vi "FPGAvi.vi"() -> ()   [LabVIEW 2009]
uses:
  Signal Options.ctl
  Sequence.ctl
  <vilib>/Platform/TimedLoop/XDataNode/XDataNode.xnode
  <vilib>/Platform/TimedLoop/XDataNode/loadlvalarms.vi
  <vilib>/Platform/TimedLoop/XDataNode/timing_clust.ctl
  <vilib>/Platform/TimedLoop/XDataNode/nitl_modes.ctl
  <vilib>/Platform/TimedLoop/XDataNode/wakeup.ctl
  <vilib>/eio/EIONode/EIONode.xnode
  <vilib>/rvi/eio/nirviEIOImplementation/nirviEIOImplementation.xnode
  <vilib>/rvi/eio/common/nirviEmuTemplateMethod_noerrors.vi
  <vilib>/rvi/eio/common/nirviEmuClasses.ctl
  <vilib>/Platform/TimedLoop/XDataNode/XDNodeRunTimeDep.lvlib
panel:
  out "t_last_chop+t_dark-t_off":u64
  out "T_last-chop + t_dark":u64
  out "T_last-chop":u64
  out "t_chop":u64
  out "Current State":T1
  in  "Memory Sequence Duration":u64=240000
  out "t_mem":u64
  in  "Repump Duration":u64
  in  "Pump Duration":u64
  in  "Trapping Duration":u64
  in  "Chopper Dark Time":u64=15200
  out "Output Trigger":bool
  out "Global Time":u64
  out "Memory Timer":u64
  in  "Time to Activate B":u64=120000
  in  "Memory Mode":T2=enum."Coherent Memory Sequence"
  in  "Optical Density Sign":bool
  in  "Optical Density - stop":u64
  in  "Optical Density - start":u64
  in  "DLCZ Sign":bool
  in  "DLCZ start":u64
  in  "DLCZ stop":u64
  in  "Generate DLCZ Pulses":bool
  in  "DLCZ Period":u32
  in  "Time to Cut B":u64=120000
  in  "Minimum Period Between Memory Sequences":u64=800000
  in  "Trigger on Slope":enum8{"either", "false-true", "true-false"}(ring)=enum."true-false"
  in  "Stop":bool
  out "Active":bool
  in  "Output Trigger Sign":bool
  in  "Signal Sign":bool
  in  "Control Sign":bool
  in  "Repetition Period":u32
  in  "Switch Trigger (Shift Decimation)":bool
  in  "Trigger Source":bool
  in  "Pulse Selection":bool=TRUE
  in  "Signal stop":u64
  in  "Control - stop":u64
  in  "Signal start":u64
  in  "Control - start":u64
  # "External"
  # "Internal"
  # "All Pulses"
  # "1 out of 2 Pulses"
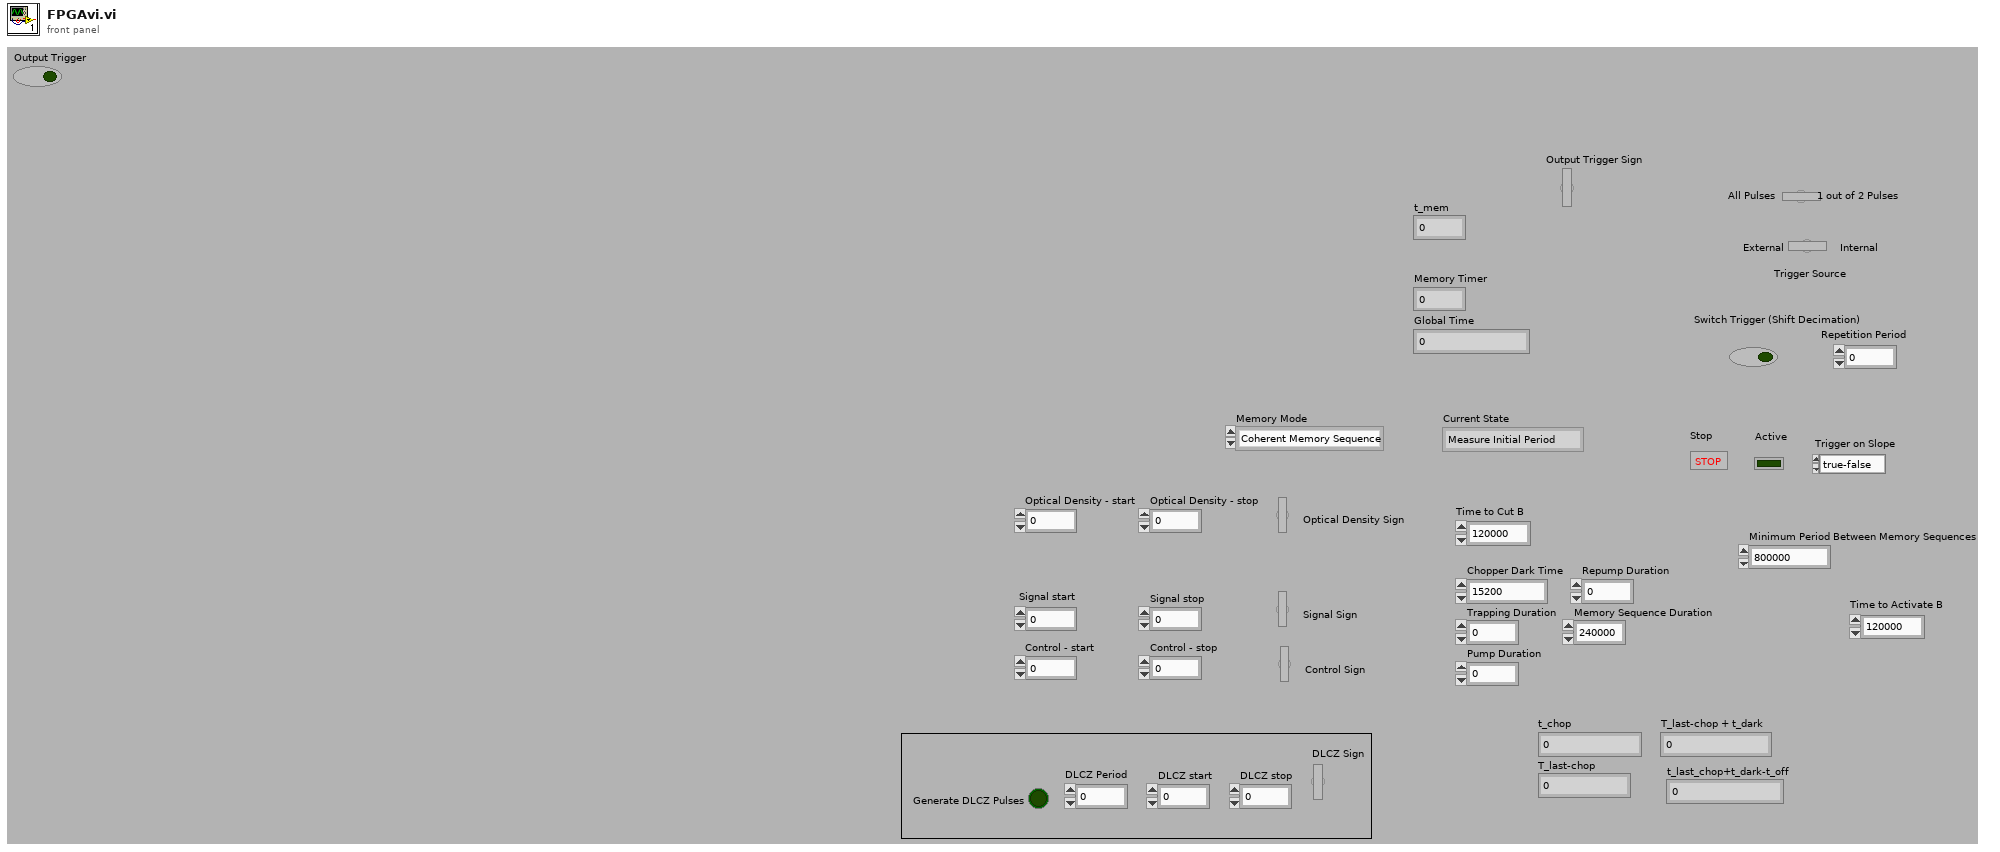
[diagram p1: front panel]
types:
  T1 = typedef "Sequence.ctl" = enum16{"Measure Initial Period", "Build MOT", "Wait for Deactivate Signal", "Deactivate B field", "Memory Sequence"}
  T2 = typedef "Signal Options.ctl" = enum16{"Generate DLCZ Pulses", "Measure Optical Density", "Coherent Memory Sequence", "Squeezed Memory Sequence"}
  T3 = typedef "XDNodeRunTimeDep.lvlib/timing_clust.ctl" = cluster{"Expected End [f-1]":u64, "Actual End [f-1]":u64, "Finished Late? [f-1]":bool, "Expected End [i-1]":u64, "Actual End [i-1]":u64, "Finished Late? [i-1]":bool, "Expected Start [i]":u64, "Actual Start [i]":u64, "Expected Start [f]":u64, "Actual Start [f]":u64, "Source Name":string, "Structure Name":string, "Period":i64, "Deadline":i64, "Offset":i64, "Start":i64, "Priority":i32, "Timeout":i32, "Mode":T4, "Wakeup Reason":T5, "Error":errorcluster, "Source Type":string, "Secondary Source Type":string, "Global End Time":u64, "Global Start Time":u64, "Frame Duration":u64, "Iteration Duration":u64, "Assigned CPU":i32, "I/O Scan Engine Mode":u32}
  T4 = typedef "XDNodeRunTimeDep.lvlib/nitl_modes.ctl" = enum32{"No Change", "Process missed periods, maintain original phase", "Discard missed periods, maintain original phase", "Process missed periods, ignore original phase", "Discard missed periods, ignore original phase"}
  T5 = typedef "XDNodeRunTimeDep.lvlib/wakeup.ctl" = enum32{"Normal", "Aborted", "Asynchronous wakeup", "Timing source error", "Timed loop error", "Timeout"}
  T6 = typedef "nirviEmuClasses.ctl" = enum16{"IO Read", "IO Write", "Method", "Property Read", "Property Write"}
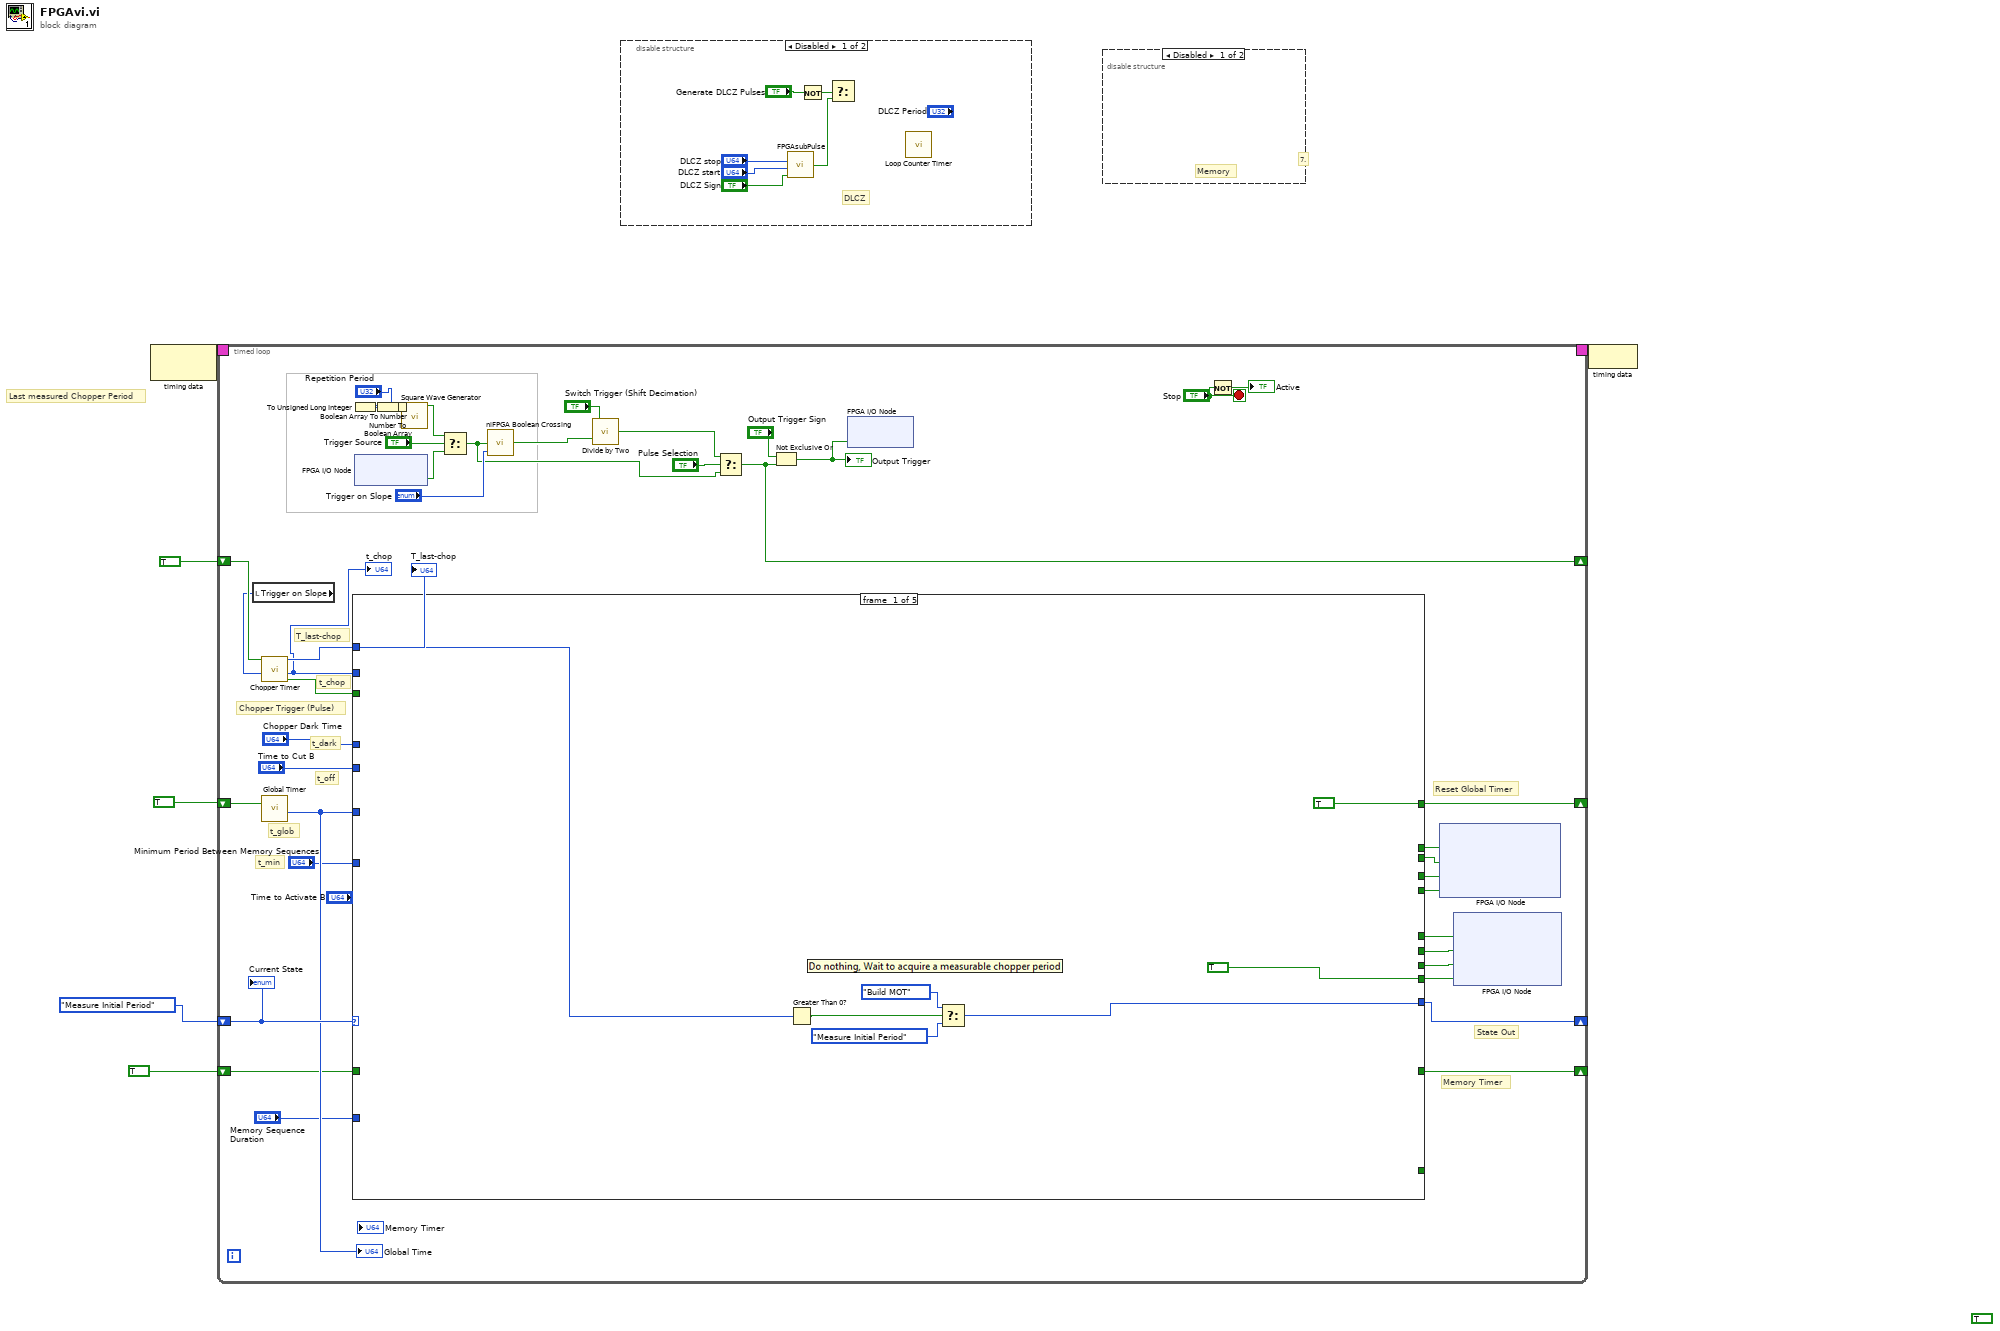
[diagram p0: block diagram]
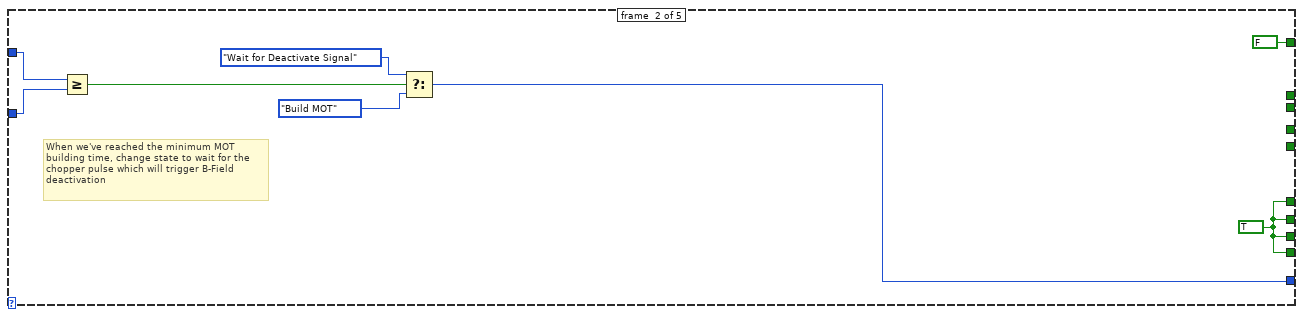
[diagram p4: hidden frame]
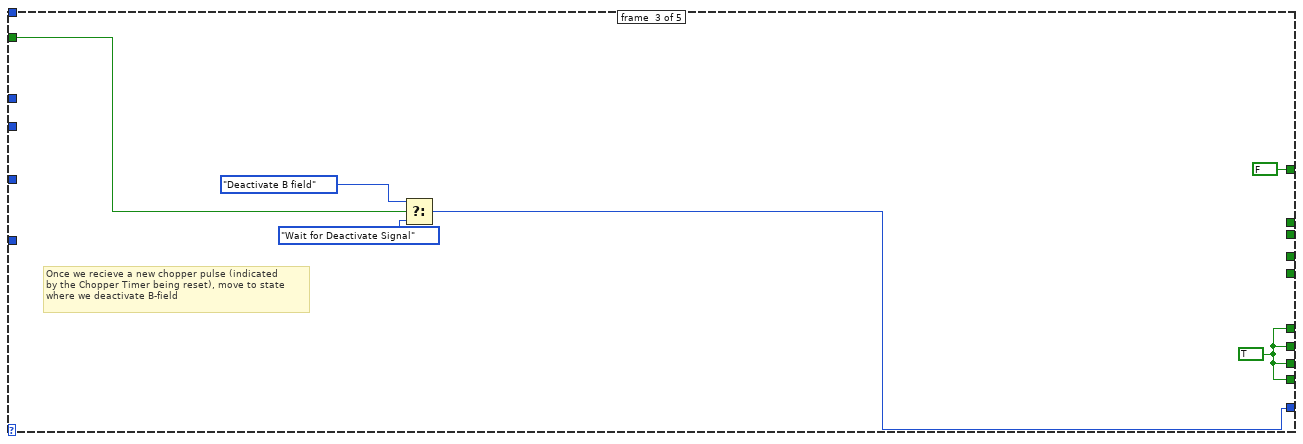
[diagram p5: hidden frame]
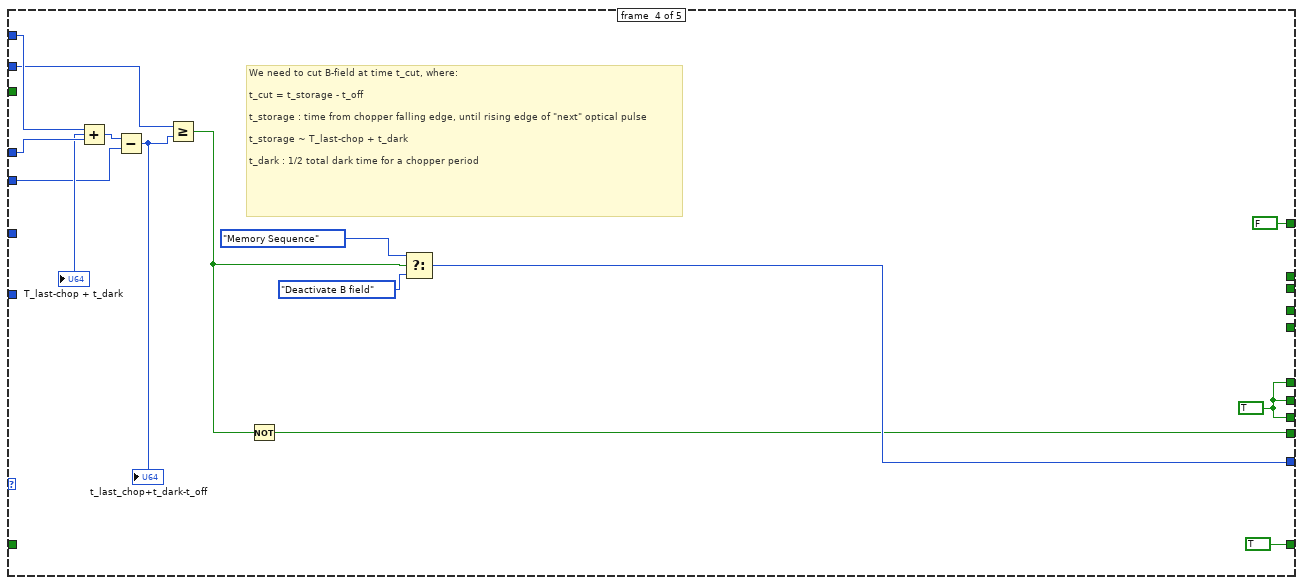
[diagram p6: hidden frame]
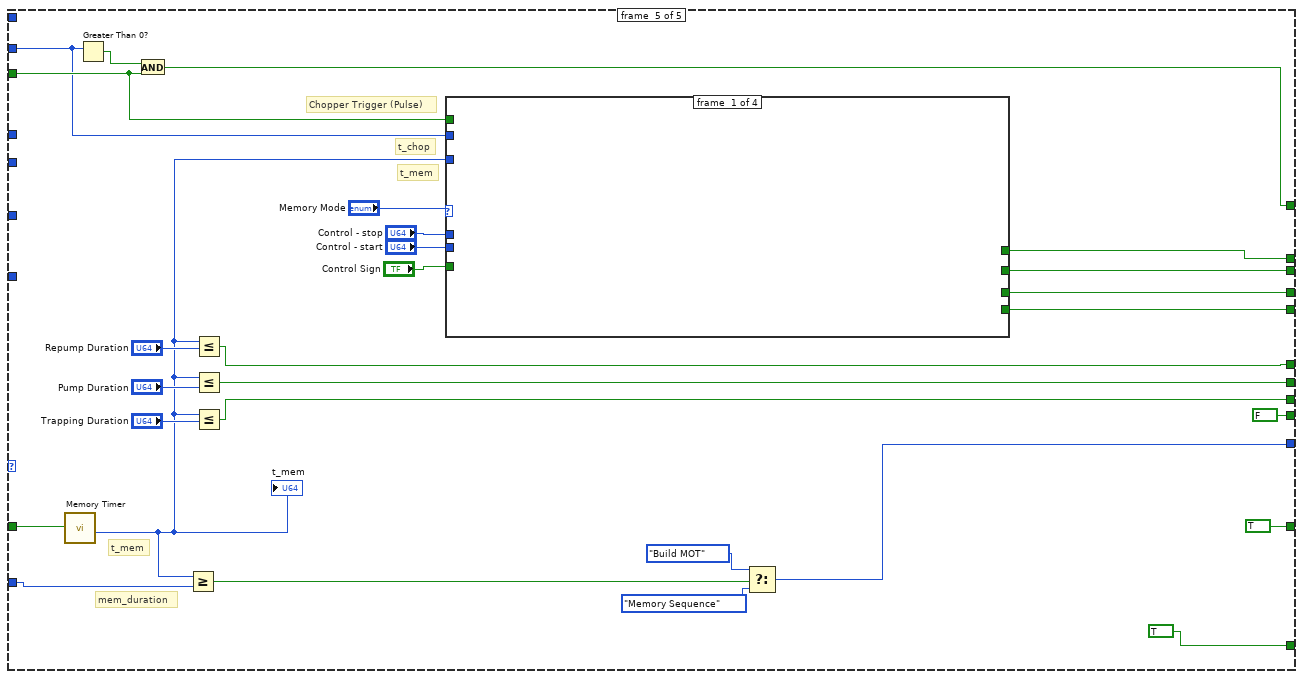
[diagram p7: hidden frame]
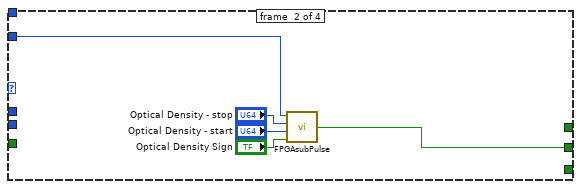
[diagram p8: hidden frame]
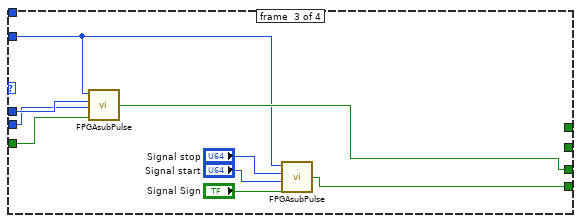
[diagram p9: hidden frame]
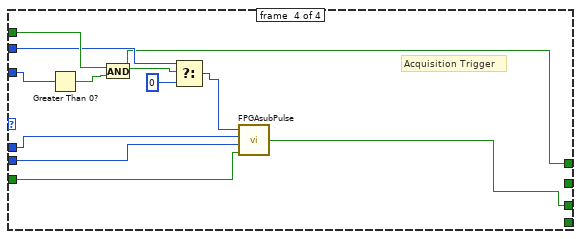
[diagram p10: hidden frame]
diagram:
  (unwired) TRUE
  # "Last measured Chopper Period"
  # "7."
  n1 = node-c288() -> (w6:T3)  [unwired: 1 out]
  n2 = timed-loop {
    timing: w6 -> [_]
    timing-out: [_] -> w5
    shift-right: [w23] -> _
    shift-left: TRUE -> [w22]
    shift-right: [w43] -> _
    shift-left: Sequence."Measure Initial Period" ("Sequence") -> [w46]
    shift-right: [w42] -> _
    shift-left: TRUE -> [w20]
    shift-right: [w13] -> _
    shift-left: TRUE -> [w12]
    stop <- "Stop" stop-if-true
    # "Memory Timer"
    # "t_dark"
    # "t_off"
    # "State Out"
    # "Reset Global Timer"
    # "t_min"
    # "Chopper Trigger (Pulse)"
    # "t_chop"
    # "T_last-chop"
    # "t_glob"
    n3 = local read "Trigger on Slope"() -> (w21:enum8{"either", "false-true", "true-false"})
    n4 = call "Chopper Timer.vi"("Trigger Direction"=w21, "Waveform"=w22) -> ("Clock Reset"=w24:bool, "Loop Counter"=w25:u64, "Last Interval between Resets"=w26:u64)  [unwired: 2 in, 1 out]
    "t_chop" <- w25
    "T_last-chop" <- w26
    n5 = call "Global Timer.vi"("Reset"=w20) -> ("Loop Counter"=w19:u64)  [unwired: 3 in, 3 out]
    "Global Time" <- w19
    n6 = To Unsigned Long Integer(number="Repetition Period") -> (unsigned 32bit integer=w31:u32)
    n7 = case shown="\"Memory Sequence\"" w46 {
      tunnel: [w127 w130 w139 w153 w183] -> w43
      tunnel: [TRUE w131 w140 w144 FALSE] -> w44
      tunnel: "Time to Cut B" -> [_ _ _ w149 _]
      tunnel: [TRUE FALSE FALSE FALSE w171] -> w42
      tunnel: w26 -> [w123 _ _ w151 _]
      tunnel: w25 -> [_ _ _ w148 w161]
      tunnel: w24 -> [_ _ w138 _ w162]
      tunnel: w19 -> [_ w136 _ _ _]
      tunnel: "Minimum Period Between Memory Sequences" -> [_ w137 _ _ _]
      tunnel: [_ w131 w140 w154 w173] -> w17
      tunnel: [_ w131 w140 w154 w174] -> w16
      tunnel: [_ w131 w140 w154 w175] -> w15
      tunnel: "Chopper Dark Time" -> [_ _ _ w152 _]
      tunnel: [_ _ _ TRUE TRUE] -> w13
      tunnel: w12 -> [_ _ _ _ w181]
      tunnel: "Memory Sequence Duration" -> [_ _ _ _ w180]
      tunnel: [_ _ _ _ w168] -> w10
      tunnel: [_ _ _ _ w167] -> w9
      tunnel: [_ _ _ _ w166] -> w8
      tunnel: [_ _ _ _ w160] -> w7
      tunnel: [_ _ _ _ TRUE] -> _
      frame #0 {
        n8 = Greater Than 0?(x=w123) -> (x > 0?=w124:bool)
        n9 = Select(t=Sequence."Build MOT" ("Sequence"), s=w124, f=Sequence."Measure Initial Period" ("Sequence")) -> (s? t:f=w127:T1)
      }
      frame #1 {
        w131 = TRUE
        # "When we've reached the minimum MOT\nbuilding time, change state to wait for the\nchopper pulse which will trigger B-Field \ndeactivation"
        n10 = Greater Or Equal?(x=w136, y=w137) -> (x >= y?=w134:bool)
        n11 = Select(t=Sequence."Wait for Deactivate Signal" ("Sequence"), s=w134, f=Sequence."Build MOT" ("Sequence")) -> (s? t:f=w130:T1)
      }
      frame #2 {
        w140 = TRUE
        # "Once we recieve a new chopper pulse (indicated \nby the Chopper Timer being reset), move to state \nwhere we deactivate B-field"
        n12 = Select(t=Sequence."Deactivate B field" ("Sequence"), s=w138, f=Sequence."Wait for Deactivate Signal" ("Sequence")) -> (s? t:f=w139:T1)
      }
      frame #3 {
        w154 = TRUE
        # "We need to cut B-field at time t_cut, where:\n\nt_cut = t_storage - t_off\n\nt_storage : time from chopper falling edge, until rising edge of \"next\" optical pulse\n\nt_storage ~ T_last-chop + t_dark\n\nt_dark : 1/2 total dark time for a chopper period"
        n13 = Add(x=w151, y=w152) -> (x+y=w150:u64)
        "T_last-chop + t_dark" <- w150
        n14 = Subtract(x=w150, y=w149) -> (x-y=w147:u64)
        "t_last_chop+t_dark-t_off" <- w147
        n15 = Greater Or Equal?(x=w148, y=w147) -> (x >= y?=w145:bool)
        n16 = Not(x=w145) -> (.not. x?=w144:bool)
        n17 = Select(t=Sequence."Memory Sequence" ("Sequence"), s=w145, f=Sequence."Deactivate B field" ("Sequence")) -> (s? t:f=w153:T1)
      }
      frame #4 {
        # "t_chop"
        # "t_mem"
        # "Chopper Trigger (Pulse)"
        # "mem_duration"
        # "t_mem"
        n18 = call "Memory Timer.vi"("Reset"=w181) -> ("Loop Counter"=w169:u64)  [unwired: 3 in, 3 out]
        "t_mem" <- w169
        n19 = Greater Than 0?(x=w161) -> (x > 0?=w172:bool)
        n20 = And(x=w172, y=w162) -> (x .and. y?=w171:bool)
        n21 = Greater Or Equal?(x=w169, y=w180) -> (x >= y?=w179:bool)
        n22 = Less Or Equal?(x=w169, y="Repump Duration") -> (x <= y?=w173:bool)
        n23 = Less Or Equal?(x=w169, y="Pump Duration") -> (x <= y?=w174:bool)
        n24 = Less Or Equal?(x=w169, y="Trapping Duration") -> (x <= y?=w175:bool)
        n25 = case shown="\"Squeezed Memory Sequence\"" "Memory Mode" {
          tunnel: w169 -> [_ w187 w191 w206]
          tunnel: [_ w186 _ _] -> w168
          tunnel: [_ _ w195 _] -> w167
          tunnel: [_ _ w196 w207] -> w166
          tunnel: "Control - stop" -> [_ _ w194 w210]
          tunnel: "Control - start" -> [_ _ w193 w209]
          tunnel: "Control Sign" -> [_ _ w192 w208]
          tunnel: w162 -> [_ _ _ w204]
          tunnel: w161 -> [_ _ _ w203]
          tunnel: [_ _ _ w200] -> w160
          frame #0 {
          }
          frame #1 {
            n26 = call "FPGAsubPulse.vi"("Signal Sign"="Optical Density Sign", "Signal start"="Optical Density - start", "Signal stop"="Optical Density - stop", "Clock"=w187) -> ("Boolean"=w186:bool)
          }
          frame #2 {
            n27 = call "FPGAsubPulse.vi"("Signal Sign"=w192, "Signal start"=w193, "Signal stop"=w194, "Clock"=w191) -> ("Boolean"=w196:bool)
            n28 = call "FPGAsubPulse.vi"("Signal Sign"="Signal Sign", "Signal start"="Signal start", "Signal stop"="Signal stop", "Clock"=w191) -> ("Boolean"=w195:bool)
          }
          frame #3 {
            # "Acquisition Trigger"
            n29 = Greater Than 0?(x=w206) -> (x > 0?=w205:bool)
            n30 = And(x=w204, y=w205) -> (x .and. y?=w200:bool)
            n31 = Select(t=w203, s=w200, f=u64 0) -> (s? t:f=w202:u64)
            n32 = call "FPGAsubPulse.vi"("Signal Sign"=w208, "Signal start"=w209, "Signal stop"=w210, "Clock"=w202) -> ("Boolean"=w207:bool)
          }
        }
        n33 = Select(t=Sequence."Build MOT" ("Sequence"), s=w179, f=Sequence."Memory Sequence" ("Sequence")) -> (s? t:f=w183:T1)
      }
    }
    n34 = xnode "FPGA I/O Node"() -> ("chopper"=w28:bool)  [unwired: 1 in, 1 out]
    n35 = Number To Boolean Array(number=w31) -> (Boolean array=w33:bool[])
    n36 = Boolean Array To Number(Boolean array=w33) -> (number=w32:fxp<+,32,0>)
    n37 = call "Square Wave Generator"("frequency (periods/tick)"=w32) -> ("square wave out"=w27:bool)  [unwired: 14 in]
    n38 = Select(t=w27, s="Trigger Source", f=w28) -> (s? t:f=w29:bool)
    n39 = call <vilib>:"niFPGA Boolean Crossing.vi"("input"=w29, "direction"="Trigger on Slope") -> ("crossing"=w30:bool)  [unwired: 1 in, 6 out]
    n40 = call "Divide by Two.vi"("Input Trigger"=w30, "Switch Trigger (Shift Decimation)"="Switch Trigger (Shift Decimation)") -> ("Decimated Trigger"=w34:bool)
    n41 = Select(t=w34, s="Pulse Selection", f=w29) -> (s? t:f=w23:bool)
    n42 = Not Exclusive Or(1:w23, 2:"Output Trigger Sign") -> (0:w35:bool)
    "Output Trigger" <- w35
    n43 = xnode "FPGA I/O Node"("trigger"=w35) -> ()  [unwired: 1 in, 1 out]
    n44 = Not(x="Stop") -> (.not. x?=→"Active":bool)
    n45 = xnode "FPGA I/O Node"("Acquisition Trigger"=w7, "Optical Density"=w10, "control"=w8, "signal"=w9) -> ()  [unwired: 4 in, 4 out]
    n46 = xnode "FPGA I/O Node"("repump"=w17, "pump"=w16, "Trapping Beams"=w15, "B-Field"=w44) -> ()  [unwired: 4 in, 4 out]
    "Current State" <- w46
  }
  n47 = disable-structure shown="Disabled" {
    frame #0 {
      # "DLCZ"
      n48 = call "FPGAsubPulse.vi"("Signal Sign"="DLCZ Sign", "Signal start"="DLCZ start", "Signal stop"="DLCZ stop") -> ("Boolean"=w262:bool)  [unwired: 1 in]
      n49 = Not(x="Generate DLCZ Pulses") -> (.not. x?=w261:bool)
      n50 = Select(s=w261, f=w262) -> ()  [unwired: 1 in, 1 out]
      n51 = call "Loop Counter Timer.vi"() -> ()  [unwired: 4 in, 4 out]
    }
    frame #1 {
    }
  }
  n52 = disable-structure shown="Disabled" {
    frame #0 {
      # "Memory"
    }
    frame #1 {
    }
  }
  n53 = node-c288(w5) -> ()
